vi "Launcher.vi"(8 "error in (no error)":errorcluster, 10 "Log Class":refnum<class "Build_Javier_Lopez_lib_Configuration_Filejson class.lvclass">, 11 "Module Launcher Base in":refnum<class "Launcher Base.lvclass">) -> (0 "error out":errorcluster)   [LabVIEW 2021, in "Launcher Base.lvclass"]
uses:
  Launcher Base.lvclass
  <vilib>/Javier Lopez/Configuration File/Json Element/Build_Javier_Lopez_lib_Configuration_Filejson class.lvclass
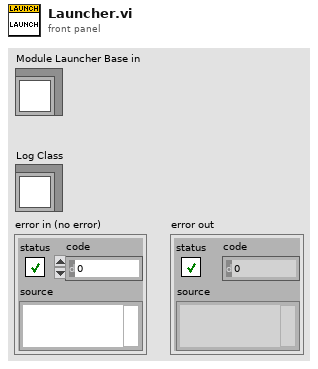
[diagram p1: front panel]
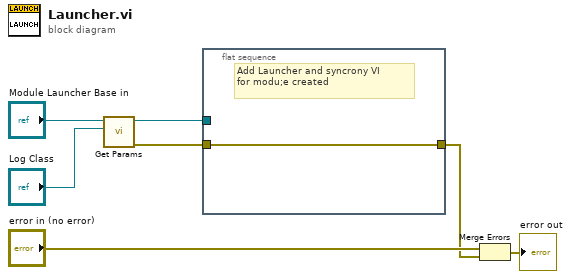
[diagram p0: block diagram]
diagram:
  n1 = call-dynamic "Get Params.vi"("Log Class"="Log Class", "Module Launcher Base in"="Module Launcher Base in") -> ("error out"=w2:errorcluster, "Module Launcher Base out"=w3:refnum<class "Launcher Base.lvclass">)  [unwired: 8 in]
  n2 = flat-sequence {
    tunnel: w3 -> [_]
    tunnel: w2 -> [w8]
    tunnel: [w8] -> w1
    frame #0 {
      # "Add Launcher and syncrony VI\nfor modu;e created"
    }
  }
  n3 = Merge Errors("error in (no error)", w1) -> (→"error out":errorcluster)
